vi "Semaphore Try Wait.vi"(8 "error in (no error)":errorcluster, 11 "Semaphore in":T1) -> (0 "error out":errorcluster, 2 "try again?":bool, 3 "Semaphore out":T1)   [LabVIEW 2013, in "POSIX Threads.lvlib" / "Semaphore.lvclass"]
doc: "Calls sem_trywait() on the semaphore object encapsulated by Semaphore.\n\nThis VI attempts to decrement the value of the semaphore by 1. If the semaphore has a value of zero, this VI returns immediately and indicates the semaphore was not set. If the sempahore has a value that is greater than zero, this function decrements the semaphore and returns indicating that it was successful in decrementing the semaphore.\n\nRefer to online POSIX documentation for more information."
uses:
  Semaphore.lvclass
  Controls/reference.ctl
  POSIX Thread Object/POSIX Thread Object.lvclass/POSIX Thread Object.ctl
  POSIX Thread Object/Private VIs/libpthread path.vi
  POSIX Thread Object/Private VIs/get pthread error.vi
  <vilib>/NI/NI Linux RT Errno/VIs/Public/SubVIs/errno enum to number.vi
  <vilib>/NI/NI Linux RT Errno/VIs/Public/Get Errno Value for Calling Thread.vi
  POSIX Thread Object/POSIX Thread Object.lvclass
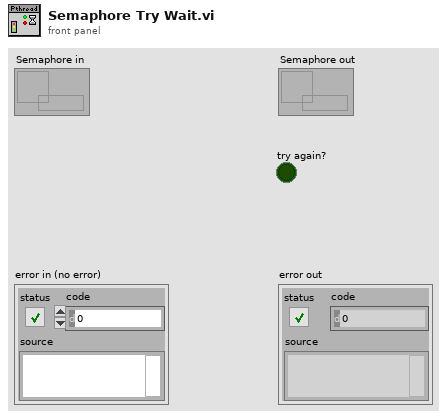
[diagram p1: front panel]
types:
  T1 = typedef "POSIX Threads.lvlib/Semaphore.lvclass/reference.ctl" = refnum<data-value>
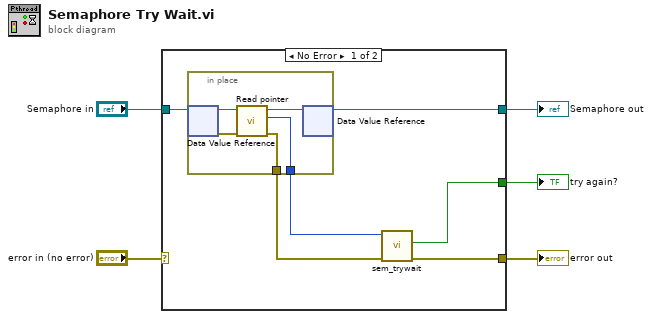
[diagram p0: block diagram]
diagram:
  n1 = case shown="No Error" "error in (no error)" {
    selector: "error in (no error)" -> [_ w17]
    tunnel: "Semaphore in" -> [w11 w18]
    tunnel: [w10 w18] -> w2
    tunnel: [w8 w17] -> w3
    tunnel: [w6 _] -> w1
    frame No Error {
      n2 = in-place {
        in-place-border: [w13] -> w9
        in-place-border: [w12] -> w7
        n3 = in-place-dvr #1(w11) -> (w16:refnum<class "Semaphore.lvclass">, w15:errorcluster)
        n4 = call "Read pointer.vi"("error in (no error)"=w15, "POSIX Thread Object in"=w16) -> ("error out"=w13:errorcluster, "pointer"=w12:u64, "POSIX Thread Object out"=w14:refnum<class "Semaphore.lvclass">)  [unwired: 7 in]
        n5 = in-place-dvr #1(w14) -> (w10:T1)  [unwired: 1 out]
      }
      n6 = call "sem_trywait.vi"("error in (no error)"=w9, "sempahore ptr in"=w7) -> ("error out"=w8:errorcluster, "try again?"=w6:bool)  [unwired: 7 in, 1 out]
    }
    frame Error {
    }
  }
  "error out" <- w3
  "Semaphore out" <- w2
  "try again?" <- w1
